vi "Get Open Time.vi"(8 "error in (no error)":errorcluster, 11 "hdl":i32) -> (0 "error out":errorcluster, 2 "Open Time":i32, 3 "hdl out":i32)   [LabVIEW 2013, in "Thorlabs_SC10.lvlib"]
doc: "Returns offset value. false represents no tune performed."
uses:
  <instrlib>/Thorlabs_SC10/Thorlabs_SC10.lvlib
  <instrlib>/Thorlabs_SC10/Data/SC10CommandLib_x64.dll
  <instrlib>/Thorlabs_SC10/Data/SC10CommandLib_win32.dll
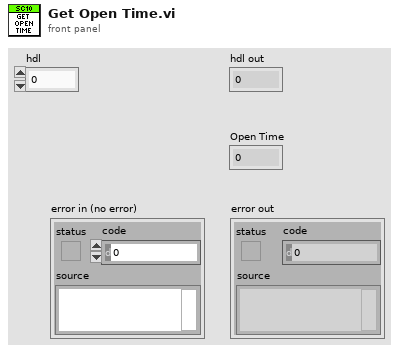
[diagram p1: front panel]
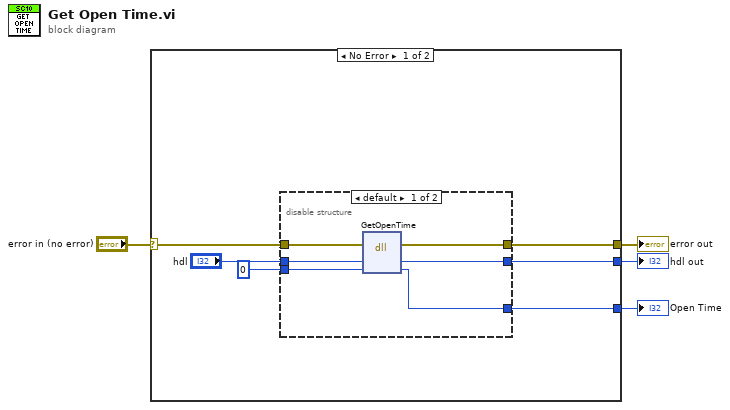
[diagram p0: block diagram]
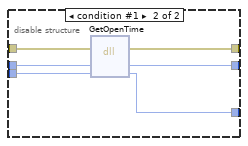
[diagram p2: hidden frame]
diagram:
  n1 = case shown="No Error" "error in (no error)" {
    selector: "error in (no error)" -> [w10 w23]
    tunnel: [w9 w23] -> w4
    tunnel: [w7 _] -> w2
    tunnel: [w8 _] -> w1
    frame No Error {
      n2 = disable-structure shown="default" {
        disable-tunnel: w10 -> [w16 w22]
        disable-tunnel: [w15 w21] -> w9
        disable-tunnel: [w14 w20] -> w8
        disable-tunnel: [w13 w19] -> w7
        disable-tunnel: "hdl" -> [w12 w18]
        disable-tunnel: 0 ("value") -> [w11 w17]
        frame condition #0 (active) {
          n3 = dll-call lib="C:/Program Files (x86)/National Instruments/LabVIEW 2013/instr.lib/Thorlabs_SC10/Data/SC10CommandLib_win32.dll" fn="GetOpenTime"(error in=w16, "hdl"=w12, "value"=w11) -> (error out=w15:errorcluster, "hdl"=w14:i32, "value"=w13:i32)  [unwired: 3 in, 1 out]
        }
        frame condition #1 {
          n4 = dll-call lib="C:/Program Files/National Instruments/LabVIEW 2013/instr.lib/Thorlabs_SC10/Data/SC10CommandLib_x64.dll" fn="GetOpenTime"(error in=w22, "hdl"=w18, "value"=w17) -> (error out=w21:errorcluster, "hdl"=w20:i32, "value"=w19:i32)  [unwired: 3 in, 1 out]
        }
      }
    }
    frame Error {
    }
  }
  "error out" <- w4
  "Open Time" <- w2
  "hdl out" <- w1
